vi "Fgen Basic Standard Function.vi"() -> ()   [LabVIEW 2021]
doc: "This example shows how to use Standard Function mode. This is a basic example that shows the smallest amount of code necessary to generate a standard waveform."
uses:
  <instrlib>/niFgen/niFgen.llb/niFgen Output Mode.ctl
panel:
  in  "Standard Waveform":u16(ring) items=["Sine", "Square", "Triangle", "Ramp Up", "Ramp Down", "DC", "Noise"]
  in  "Stop":bool
  in  "FGEN Resource Name":refnum<k15>="PXI1Slot3"
  in  "Frequency":dbl=1000000.0 format="%.2p"
  in  "Amplitude":dbl=2.0 format="%0_3g"
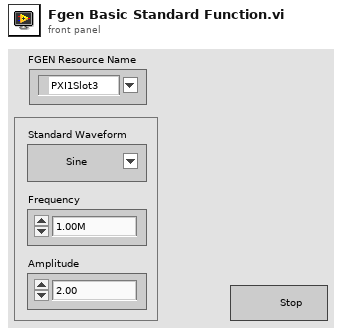
[diagram p1: front panel]
types:
  T1 = typedef "niFgen Output Mode.ctl" = u32
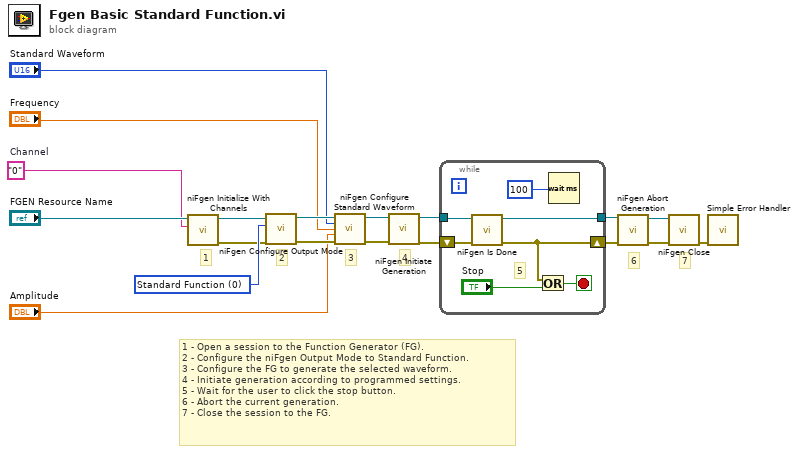
[diagram p0: block diagram]
diagram:
  w1 = "0"  # Channel
  w17 = T1 0 items=["Standard Function", "Frequency List", "Arbitrary Waveform", "Arbitrary Sequence", "Script"] ("output mode")
  # "7"
  # "6"
  # "4"
  # "3"
  # "2"
  # "1"
  # "1 - Open a session to the Function Generator (FG).\n2 - Configure the niFgen Output Mode to Standard Function.\n3 - Configure the FG to generate the selected waveform.\n4 - Initiate generation according to programmed settings.\n5 - Wait for the user to click the stop button.\n6 - Abort the current generation.\n7 - Close the session to the FG."
  n1 = call <instrlib>:"niFgen Initialize With Channels.vi"("Channel Name"=w1, "Resource Name"="FGEN Resource Name") -> ("error out"=w2:errorcluster, "Instrument Handle Out"=w3:refnum<k15>)  [unwired: 8 in]
  n2 = call <instrlib>:"niFgen Configure Output Mode.vi"("error in (no error)"=w2, "Output Mode (default: 0=Standard Function)"=w17, "Instrument Handle"=w3) -> ("error out"=w13:errorcluster, "Instrument Handle Out"=w14:refnum<k15>)  [unwired: 6 in]
  n3 = call <instrlib>:"niFgen Configure Standard Waveform.vi"("Instrument Handle"=w14, "Waveform"="Standard Waveform", "Frequency"="Frequency", "Amplitude"="Amplitude", "error in (no error)"=w13) -> ("Instrument Handle Out"=w15:refnum<k15>, "error out"=w16:errorcluster)  [unwired: 9 in]
  n4 = call <instrlib>:"niFgen Initiate Generation.vi"("error in (no error)"=w16, "Instrument Handle"=w15) -> ("error out"=w18:errorcluster, "Instrument Handle Out"=w19:refnum<k15>)  [unwired: 8 in]
  n5 = while {
    tunnel: w19 -> [w22]
    tunnel: [w21] -> w10
    shift-right: [w20] -> w12
    shift-left: w18 -> [w23]
    stop <- w25 stop-if-true
    # "5"
    # "Wait for User \nto hit Stop"
    n6 = call <instrlib>:"niFgen Is Done.vi"("error in (no error)"=w23, "Instrument Handle"=w22) -> ("error out"=w20:errorcluster, "Instrument Handle Out"=w21:refnum<k15>)  [unwired: 7 in, 1 out]
    n7 = Or(x=w20, y="Stop") -> (x .or. y?=w25:bool)
    n8 = Wait (ms)(milliseconds to wait=u32 100 ("millisecond multiple")) -> ()  [unwired: 1 out]
  }
  n9 = call <instrlib>:"niFgen Abort Generation.vi"("error in (no error)"=w12, "Instrument Handle"=w10) -> ("error out"=w11:errorcluster, "Instrument Handle Out"=w9:refnum<k15>)  [unwired: 8 in]
  n10 = call <instrlib>:"niFgen Close.vi"("error in (no error)"=w11, "Instrument Handle"=w9) -> ("error out"=w5:errorcluster)  [unwired: 9 in]
  n11 = call <vilib>:"Simple Error Handler.vi"("error in (no error)"=w5) -> ()  [unwired: 4 in, 5 out]
